vi "電動回転ステージプログラムver.1.1.vi"() -> ()   [LabVIEW 2020]
uses:
  Thorlabs.MotionControl.TCube.DCServoCLI.dll
  Thorlabs.MotionControl.Controls.dll
panel:
  in  "ミリ秒待機時間":u32
  in  "停止 2":bool
  in  "End Position":dbl
  in  "Step Size":dbl
  out "GetPositionCounter":sgl
  in  "停止":bool
  in  "SerialNumber":string="83862739"
  in  "TCubeDCServoControl":refnum<k24>(container)
  # "電動回転ステージ"
  # "Kinesisコントロールエリア"
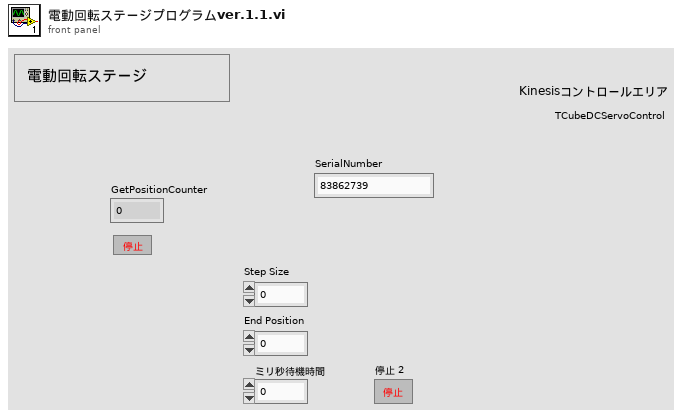
[diagram p1: front panel]
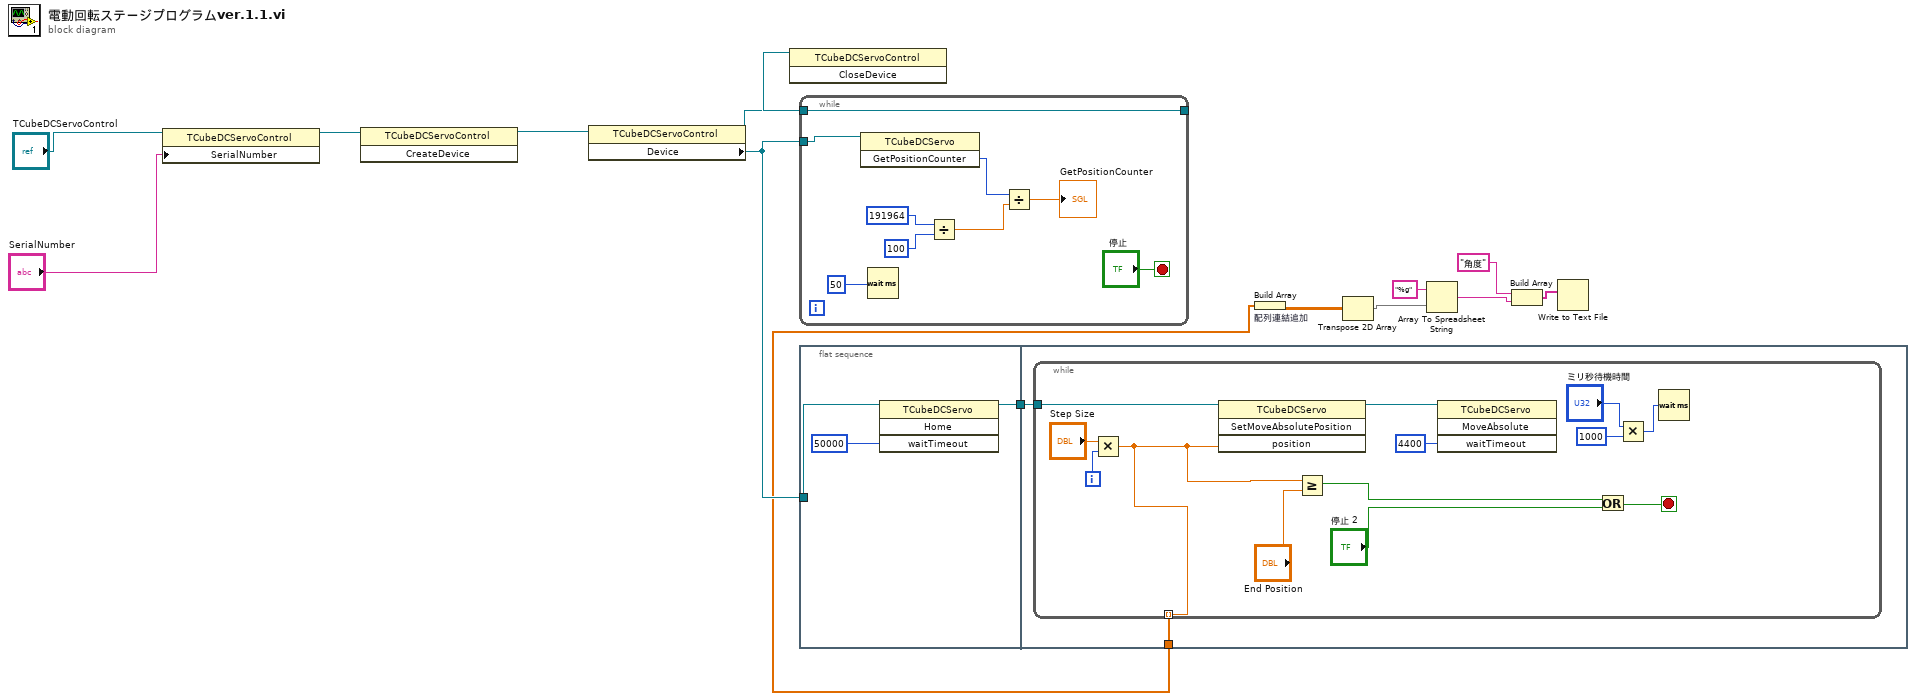
[diagram p0: block diagram]
diagram:
  n1 = property on="プロパティノード" class="TCubeDCServoControl"(reference="TCubeDCServoControl", "SerialNumber"="SerialNumber") -> (reference out=w14:refnum<k24>)  [unwired: 1 in, 1 out]
  n2 = invoke on="インボークノード" class="TCubeDCServoControl" method="CreateDevice"(reference=w14) -> (reference out=w12:refnum<k24>)  [unwired: 2 in, 2 out]
  n3 = property class="TCubeDCServoControl"(reference=w12) -> (reference out=w11:refnum<k24>, "Device"=w8:refnum<k24>)  [unwired: 1 in, 1 out]
  n4 = while {
    tunnel: [w23] -> w13
    tunnel: w11 -> [w23]
    tunnel: w8 -> [w18]
    stop <- "停止" stop-if-true
    n5 = invoke class="TCubeDCServo" method="GetPositionCounter"(reference=w18) -> ("GetPositionCounter"=w17:i32)  [unwired: 2 in, 2 out]
    n6 = Wait (ms)(milliseconds to wait=u32 50 ("ミリ秒タイマ値")) -> ()  [unwired: 1 out]
    n7 = Divide(x=191964, y=100) -> (x/y=w19:dbl)
    n8 = Divide(x=w17, y=w19) -> (x/y=→"GetPositionCounter":dbl)
  }
  n9 = invoke on="インボークノード" class="TCubeDCServoControl" method="CloseDevice"(reference=w13) -> ()  [unwired: 2 in, 3 out]
  n10 = flat-sequence {
    tunnel: w8 -> [w27]
    tunnel: [w25] -> w10
    tunnel: w10 -> [w29]
    tunnel: [w28] -> w3
    frame #0 {
      n11 = invoke class="TCubeDCServo" method="Home"(reference=w27, "waitTimeout"=50000) -> (reference out=w25:refnum<k24>)  [unwired: 2 in, 3 out]
    }
    frame #1 {
      n12 = while {
        tunnel: w29 -> [w42]
        tunnel: [w30] -> w28 mode=indexing
        i -> [w34]
        stop <- w37 stop-if-true
        n13 = Multiply(x="Step Size", y=w34) -> (x*y=w30:dbl)
        n14 = invoke class="TCubeDCServo" method="SetMoveAbsolutePosition"(reference=w42, "position"=w30) -> (reference out=w41:refnum<k24>)  [unwired: 2 in, 3 out]
        n15 = Greater Or Equal?(x=w30, y="End Position") -> (x >= y?=w39:bool)
        n16 = invoke class="TCubeDCServo" method="MoveAbsolute"(reference=w41, "waitTimeout"=4400) -> ()  [unwired: 2 in, 4 out]
        n17 = Or(x=w39, y="停止 2") -> (x .or. y?=w37:bool)
        n18 = Multiply(x="ミリ秒待機時間", y=u32 1000) -> (x*y=w32:u32)
        n19 = Wait (ms)(milliseconds to wait=w32) -> ()  [unwired: 1 out]
      }
    }
  }
  n20 = Build Array "配列連結追加"(w3) -> (w1:dbl[][])
  n21 = Transpose 2D Array(2D array=w1) -> (transposed array=w2:dbl[][])
  n22 = Array To Spreadsheet String(array=w2, 3:"%g" ("形式文字列")) -> (spreadsheet string=w6:string)  [unwired: 1 in]
  n23 = Build Array("角度" ("要素"), w6) -> (w7:string[])
  n24 = Write to Text File(text=w7) -> ()  [unwired: 3 in, 3 out]
